vi "intWaveMA.vi"(8 "expFactor":i8=-4, 11 "ortInput":T1) -> (3 "ortOutput":T1, 4 "outputValid":bool)   [LabVIEW 2016]
uses:
  <vilib>/rvi/Memory/Memory_Emulation/nirvimemoryFastEmulation.vi
  <vilib>/rvi/Memory/Memory_Emulation/nirvimemoryEmulation.vi
  <vilib>/rvi/Emulation/niFpgaEmulationIsFPGAContextNoSignature.vi
  <vilib>/rvi/DataTransferAndStorage/Container/Common/niFpgaContainerGetUniqueNameForEmu.vi
  <vilib>/rvi/Emulation/niFpgaProcessEmulError.vi
  <vilib>/rvi/Emulation/niFpgaSctlEmulationGetInTimedLoop.vi
  <vilib>/rvi/errors/nirviReportUnexpectedCaseInternalError (U32).vi
  <vilib>/rvi/DataTransferAndStorage/Container/XNode/niFpgaContainer.xnode
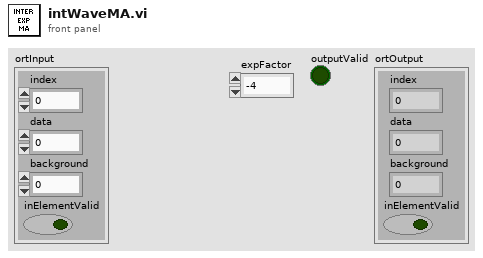
[diagram p1: front panel]
types:
  T1 = cluster{"index":u16, "data":i16, "background":i16, "inElementValid":bool}
  T2 = cluster{"index":u16, "carryOut":fxp<+/-,22,16>, "background":i16, "outputValid":bool}
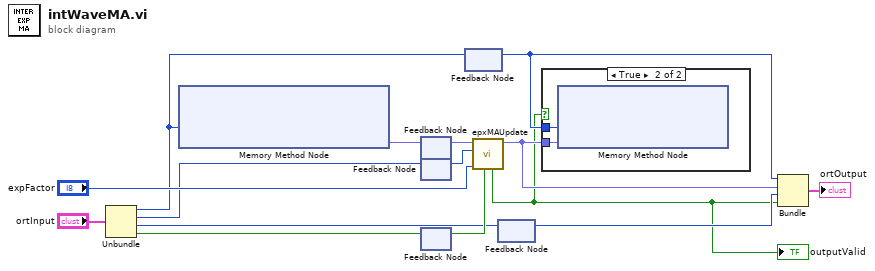
[diagram p0: block diagram]
diagram:
  n1 = Unbundle("ortInput") -> ("index"=w10:u16, "data"=w7:i16, "background"=w4:i16, "inElementValid"=w9:bool)
  n2 = xnode ("Memory Method Node")("Address"=w10) -> ("Data"=w15:fxp<+/-,22,16>)  [unwired: 1 in, 1 out]
  n3 = feedback-in #1(w15) -> ()
  n4 = feedback #1() -> (w14:fxp<+/-,22,16>)  [unwired: 1 in]
  n5 = feedback-in #2(w7) -> ()
  n6 = feedback #2() -> (w12:i16)  [unwired: 1 in]
  n7 = feedback-in #3(w9) -> ()
  n8 = feedback #3() -> (w8:bool)  [unwired: 1 in]
  n9 = feedback-in #4(w10) -> ()
  n10 = feedback #4() -> (w2:u16)  [unwired: 1 in]
  n11 = call "epxMAUpdate.vi"("inputValid"=w8, "expFactor"="expFactor", "update"=w12, "carryIn"=w14) -> ("carryOut"=w5:fxp<+/-,22,16>, "outputValid"=w1:bool)  [unwired: 6 in]
  "outputValid" <- w1
  n12 = feedback #5() -> (w3:i16)  [unwired: 1 in]
  n13 = feedback-in #5(w4) -> ()
  n14 = case shown="True" w1 {
    tunnel: w2 -> [_ w17]
    tunnel: w5 -> [_ w16]
    frame False {
    }
    frame True {
      n15 = xnode ("Memory Method Node")("Address"=w17, "Data"=w16) -> ()  [unwired: 1 in, 1 out]
    }
  }
  n16 = Bundle("index"=w2, "carryOut"=w5, "background"=w3, "outputValid"=w1) -> (→"ortOutput":T2)  [unwired: 1 in]
